vi "subsetTxRxParameters.vi"(0 "Tx /Rx Settings":T1={"USRP IP Address"="192.168.11.4", "IQ Sampling\nRate [S/sec]"=10000000.0, "Carrier Frequency [Hz]"=87000000.0, "Start Trigger Time"={"whole seconds"=0, "fractional seconds"=0.0}, "Per Device"=[]} {"Per Device"."gain" format="%#_6f"; "Carrier Frequency [Hz]" min=50000000.0 max=6000000000.0 step=1000.0 format="%#.15p"; "IQ Sampling\nRate [S/sec]" format="%#_6p"}, 11 "error in (no error)":errorcluster) -> (4 "Tx /Rx  Settings (out)":T1={"USRP IP Address"="192.168.11.4", "IQ Sampling\nRate [S/sec]"=10000000.0, "Carrier Frequency [Hz]"=87000000.0, "Start Trigger Time"={"whole seconds"=0, "fractional seconds"=0.0}, "Per Device"=[]} {"Per Device"."gain" format="%#_6f"; "Carrier Frequency [Hz]" min=50000000.0 max=6000000000.0 step=1000.0 format="%#.15p"; "IQ Sampling\nRate [S/sec]" format="%#_6p"}, 15 "error out":errorcluster)   [LabVIEW 2011]
uses:
  usrpHardwareSettings.ctl
  <instrlib>/niUSRP/niUSRP Timestamp.ctl
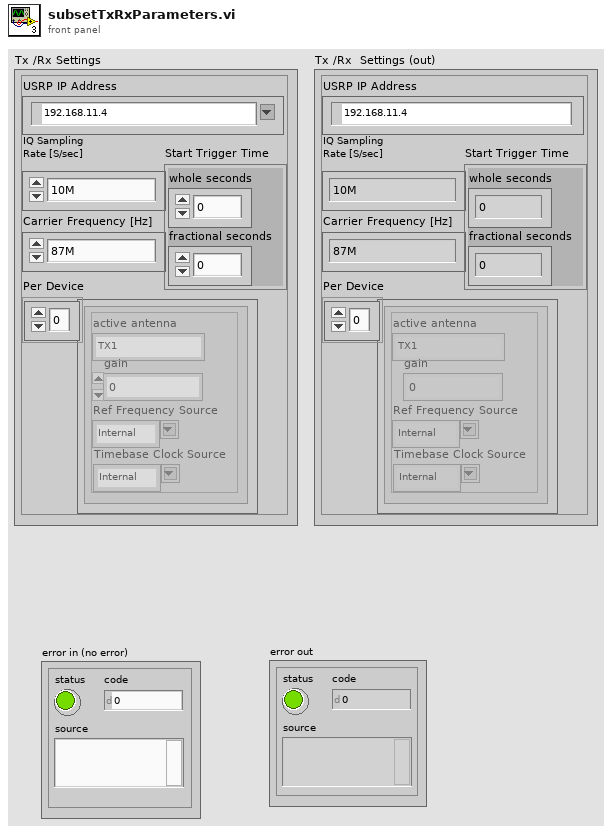
[diagram p1: front panel]
types:
  T1 = typedef "usrpHardwareSettings.ctl" = cluster{"USRP IP Address":refnum<k15>, "IQ Sampling\nRate [S/sec]":dbl, "Carrier Frequency [Hz]":dbl, "Start Trigger Time":T2, "Per Device":cluster{"active antenna":string, "gain":dbl, "Ref Frequency Source":string, "Timebase Clock Source":string}[]}
  T2 = typedef "niUSRP Timestamp.ctl" = cluster{"whole seconds":u64, "fractional seconds":dbl}
  T3 = cluster{"active antenna":string, "gain":dbl, "Ref Frequency Source":string, "Timebase Clock Source":string}[]
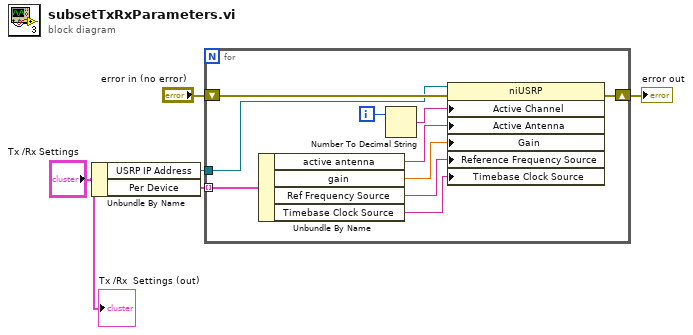
[diagram p0: block diagram]
diagram:
  n1 = Unbundle By Name("Tx /Rx Settings") -> ("USRP IP Address"=w3:refnum<k15>, "Per Device"=w1:T3)
  n2 = for {
    shift-right: [w12] -> w5
    shift-left: "error in (no error)" -> [w13]
    tunnel: w3 -> [w11]
    tunnel: w1 -> [w10] mode=indexing
    i -> [w15]
    n3 = Unbundle By Name(w10) -> ("active antenna"=w9:string, "gain"=w8:dbl, "Ref Frequency Source"=w7:string, "Timebase Clock Source"=w6:string)
    n4 = Number To Decimal String(number=w15) -> (decimal integer string=w14:string)  [unwired: 1 in]
    n5 = property class="niUSRP"(reference=w11, error in=w13, "Active Channel"=w14, "Active Antenna"=w9, "Gain"=w8, "Reference Frequency Source"=w7, "Timebase Clock Source"=w6) -> (error out=w12:errorcluster)  [unwired: 1 out]
  }
  "error out" <- w5
  "Tx /Rx  Settings (out)" <- "Tx /Rx Settings"
